vi "Test Received File Generation When Test Fails.vi"(11 "Test Case In":refnum<class "Basic Mechanics Tests.lvclass">) -> (0 "error out":errorcluster, 3 "Test Case Out":refnum<class "Basic Mechanics Tests.lvclass">)   [LabVIEW 2020, in "Basic Mechanics Tests.lvclass"]
uses:
  Basic Mechanics Tests.lvclass
  Source/Approval Tests/Options/Options.lvclass
  Source/Approval Tests/Report Nothing/Report Nothing.lvclass
  Source/Approval Tests/Scrubber/Scrubber.lvclass
  Source/Approval Tests/Namer/Namer.lvclass
  Source/Approval Tests/Naming Data/Naming Data.lvclass
  Source/Approval Tests/Reporter/Reporter.lvclass
  Source/Approval Tests/Text Comparator/Text Comparator.lvclass
  Basic Mechanics Tests.lvclass/Basic Mechanics Tests.ctl
  4be351cf-9afa-44a9-9686-c31d6937e1da.vi
  <vilib>/Astemes/LUnit/Test Case.lvclass
  5b6af433-73f2-478c-ac60-49e9a84e5db2.vi
  fbf3a6f1-25d3-4b1a-9ed1-fe282719be7b.vi
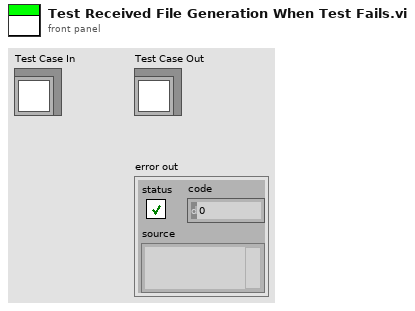
[diagram p1: front panel]
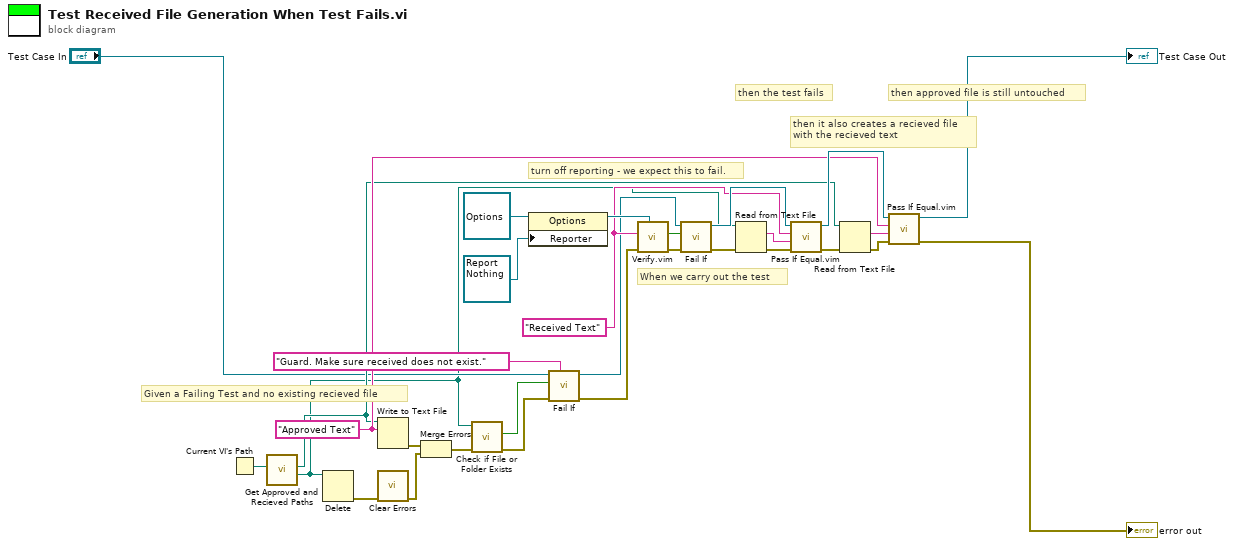
[diagram p0: block diagram]
diagram:
  w9 = "Approved Text"
  w13 = "Received Text"
  # "then approved file is still untouched"
  # "then it also creates a recieved file\nwith the recieved text"
  # "then the test fails"
  # "When we carry out the test"
  # "Given a Failing Test and no existing recieved file"
  # "turn off reporting - we expect this to fail."
  n1 = Current VI's Path() -> (path=w7:path)
  n2 = call "Get Approved and Recieved Paths.vi"("This VI"=w7) -> ("Recieved"=w3:path, "Approved Path"=w6:path)  [unwired: 9 in]
  n3 = Delete(path (use dialog)=w3) -> (error out=w30:errorcluster)  [unwired: 4 in, 2 out]
  n4 = Write to Text File(file (use dialog)=w6, text=w9) -> (error out=w29:errorcluster)  [unwired: 2 in, 2 out]
  n5 = call <vilib>:"Clear Errors.vi"("error in (no error)"=w30) -> ("error out"=w28:errorcluster)  [unwired: 5 in, 1 out]
  n6 = Merge Errors(w29, w28) -> (w27:errorcluster)
  n7 = call <vilib>:"Check if File or Folder Exists.vi"("error in (no error)"=w27, "path"=w3) -> ("error out"=w19:errorcluster, "file or folder exists?"=w2:bool)  [unwired: 7 in, 1 out]
  n8 = property on="Property Node" class="Options"(reference=refnum<class "Options.lvclass"> refnum ("Options"), "Reporter"=refnum<class "Report Nothing.lvclass"> refnum ("Approval Tests.lvlib:Report Nothing")) -> (reference out=w17:refnum<class "Options.lvclass">)  [unwired: 1 in, 1 out]
  n9 = call <vilib>:"Fail If.vi"("Description"="Guard. Make sure received does not exist.", "error in (no error)"=w19, "Fail?"=w2, "LUnit Test Case In"="Test Case In") -> ("error out"=w20:errorcluster, "LUnit Test Case Out"=w4:refnum<class "Basic Mechanics Tests.lvclass">)  [unwired: 6 in]
  n10 = call "Verify.vim"("Options"=w17, "error in"=w20, "Anything"=w13) -> ("error out"=w23:errorcluster, "Passed?"=w15:bool)  [unwired: 6 in, 1 out]
  n11 = call <vilib>:"Fail If.vi"("error in (no error)"=w23, "Fail?"=w15, "LUnit Test Case In"=w4) -> ("error out"=w22:errorcluster, "LUnit Test Case Out"=w14:refnum<class "Basic Mechanics Tests.lvclass">)  [unwired: 7 in]
  n12 = Read from Text File(file (use dialog)=w3, error in=w22) -> (text=w12:string, error out=w21:errorcluster)  [unwired: 2 in, 2 out]
  n13 = call "Pass If Equal.vim"("error in (no error)"=w21, "Actual"=w12, "Expected"=w13, "LUnit Test Case In"=w14) -> ("error out"=w24:errorcluster, "LUnit Test Case Out"=w11:refnum<class "Basic Mechanics Tests.lvclass">)  [unwired: 6 in]
  n14 = Read from Text File(file (use dialog)=w6, error in=w24) -> (text=w8:string, error out=w25:errorcluster)  [unwired: 2 in, 2 out]
  n15 = call "Pass If Equal.vim"("error in (no error)"=w25, "Actual"=w8, "Expected"=w9, "LUnit Test Case In"=w11) -> ("error out"=→"error out":errorcluster, "LUnit Test Case Out"=→"Test Case Out":refnum<class "Basic Mechanics Tests.lvclass">)  [unwired: 6 in]
